vi "Change coord.vi"(1 "Principal Planes":dbl[][](array[numeric]) format="%.2f", 2 "Angle":dbl=-45.0) -> (0 "New Planes":dbl[][](array[numeric]) format="%.2f")   [LabVIEW 2013]
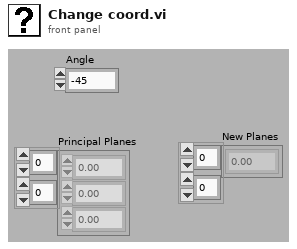
[diagram p1: front panel]
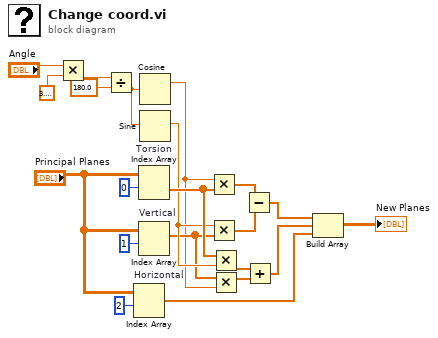
[diagram p0: block diagram]
diagram:
  n1 = Multiply(x="Angle", y=3.141592653589793) -> (x*y=w13:dbl)
  n2 = Divide(x=w13, y=180.0) -> (x/y=w11:dbl)
  n3 = Index Array "Horizontal"(array="Principal Planes", index (row)=2 ("Index (row)")) -> (element=w17:dbl[])  [unwired: 1 in]
  n4 = Index Array "Torsion"(array="Principal Planes", index (row)=0 ("Index (row)")) -> (element=w7:dbl[])  [unwired: 1 in]
  n5 = Index Array "Vertical"(array="Principal Planes", index (row)=1 ("Index (row)")) -> (element=w5:dbl[])  [unwired: 1 in]
  n6 = Cosine(x=w11) -> (cos(x)=w4:dbl)
  n7 = Sine(x=w11) -> (sin(x)=w6:dbl)
  n8 = Multiply(x=w4, y=w7) -> (x*y=w10:dbl[])
  n9 = Multiply(x=w6, y=w5) -> (x*y=w8:dbl[])
  n10 = Multiply(x=w7, y=w6) -> (x*y=w3:dbl[])
  n11 = Multiply(x=w5, y=w4) -> (x*y=w2:dbl[])
  n12 = Subtract(x=w10, y=w8) -> (x-y=w9:dbl[])
  n13 = Add(x=w3, y=w2) -> (x+y=w1:dbl[])
  n14 = Build Array(w9, w1, w17) -> (→"New Planes":dbl[][])
